vi "Constants.vi"() -> ()   [LabVIEW 2020, in "PXI-2512 Shared.lvlib"]
doc: "Use this Global VI to access the GUIDs assigned to the page resources of the Custom Device."
uses:
  PXI-2512 Shared.lvlib
panel:
  in  "Tab Control":enum32{"GUIDs", "Constants", "Properties"}(tab)
  in  "Disable PXI-2512 GUID":string="02ae7a20-0517-4abc-b4c5-b9f23f35dfb4"
  in  "PXI-2512 Channel Page":string="bca8f785-819d-40ff-83e0-8d327021cf84"
  in  "PXI-2512":string="36055fd0-ddc2-41cd-bbbe-88f7bb62b48e"
  in  "Fault Channel Description":string="The \"Name (Alias)\" for each channel may be changed. The \"Hardware Channel #\" cannot be changed by the user, and represents the actual Fault Channel being controller.\n\nThe Fault Default Value sets the default state for the channel."
  in  "Channel Fault":string="Channel Fault"
  in  "FIU Description":string="This is a Custom Device for the PXI-2512 FIU."
  in  "Hardware Device Name":string="Hardware Device Name"
  in  "FIU Channel #":string="FIU Channel #"
  in  "Compiled.Settings":string="Compiled.Settings"
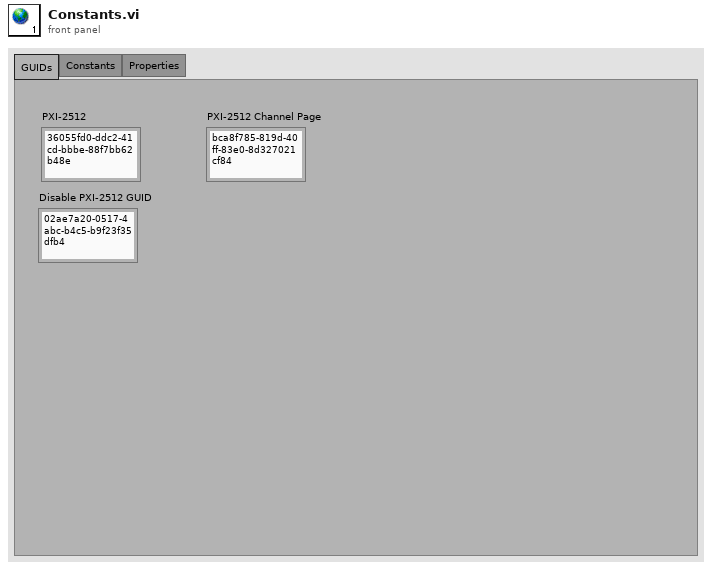
[diagram p1: front panel]
diagram:
